vi "43 Config File Get Input Scales (x64-2018).vi"   [LabVIEW 2017]
uses:
  <vilib>/Utility/config.llb/Read Key (I32).vi
  24 Global Front Panel (x64-2018).vi
  <vilib>/Utility/config.llb/NI_LVConfig.lvlib
types:
  T1 = typedef "NI_LVConfig.lvlib/Config Data RefNum.ctl" = refnum<k1>
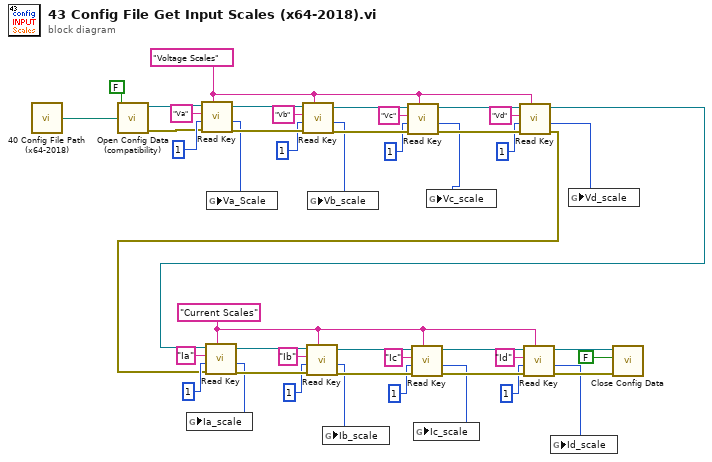
[diagram p0: block diagram]
diagram:
  w15 = "Current Scales" ("section")
  w16 = "Voltage Scales" ("section")
  n1 = call "40 Config File Path (x64-2018).vi"() -> ("Configuration File Path"=w9:path)
  n2 = call <vilib>:"Open Config Data (compatibility).vi"("create file if necessary (T)"=FALSE ("create file if necessary? (T)"), "configuration file path"=w9) -> ("error out"=w33:errorcluster, "refnum"=w32:T1)  [unwired: 7 in, 1 out]
  n3 = call-poly <vilib>:"Read Key.vi"("section"=w16, "error in (no error)"=w33, "default value"=1, "key"="Va", "refnum"=w32) -> ("error out"=w39:errorcluster, "value"=w8:i32, "refnum out"=w38:T1)  [unwired: 3 in, 1 out]
  n4 = global write "24 Global Front Panel (x64-2018).vi" "Va_Scale"(w8) -> ()
  n5 = call-poly <vilib>:"Read Key.vi"("section"=w16, "error in (no error)"=w39, "default value"=1, "key"="Vb", "refnum"=w38) -> ("error out"=w43:errorcluster, "value"=w7:i32, "refnum out"=w42:T1)  [unwired: 3 in, 1 out]
  n6 = global write "24 Global Front Panel (x64-2018).vi" "Vb_scale"(w7) -> ()
  n7 = call-poly <vilib>:"Read Key.vi"("section"=w16, "error in (no error)"=w43, "default value"=1, "key"="Vc", "refnum"=w42) -> ("error out"=w47:errorcluster, "value"=w6:i32, "refnum out"=w46:T1)  [unwired: 3 in, 1 out]
  n8 = global write "24 Global Front Panel (x64-2018).vi" "Vc_scale"(w6) -> ()
  n9 = call-poly <vilib>:"Read Key.vi"("section"=w16, "error in (no error)"=w47, "default value"=1, "key"="Vd", "refnum"=w46) -> ("error out"=w10:errorcluster, "value"=w5:i32, "refnum out"=w17:T1)  [unwired: 3 in, 1 out]
  n10 = call-poly <vilib>:"Read Key.vi"("section"=w15, "error in (no error)"=w10, "default value"=1, "key"="Ia", "refnum"=w17) -> ("error out"=w23:errorcluster, "value"=w4:i32, "refnum out"=w22:T1)  [unwired: 3 in, 1 out]
  n11 = global write "24 Global Front Panel (x64-2018).vi" "Ia_scale"(w4) -> ()
  n12 = call-poly <vilib>:"Read Key.vi"("section"=w15, "error in (no error)"=w23, "default value"=1, "key"="Ib", "refnum"=w22) -> ("error out"=w27:errorcluster, "value"=w3:i32, "refnum out"=w26:T1)  [unwired: 3 in, 1 out]
  n13 = global write "24 Global Front Panel (x64-2018).vi" "Ib_scale"(w3) -> ()
  n14 = call-poly <vilib>:"Read Key.vi"("section"=w15, "error in (no error)"=w27, "default value"=1, "key"="Ic", "refnum"=w26) -> ("error out"=w31:errorcluster, "value"=w2:i32, "refnum out"=w30:T1)  [unwired: 3 in, 1 out]
  n15 = global write "24 Global Front Panel (x64-2018).vi" "Ic_scale"(w2) -> ()
  n16 = call-poly <vilib>:"Read Key.vi"("section"=w15, "error in (no error)"=w31, "default value"=1, "key"="Id", "refnum"=w30) -> ("error out"=w13:errorcluster, "value"=w1:i32, "refnum out"=w14:T1)  [unwired: 3 in, 1 out]
  n17 = global write "24 Global Front Panel (x64-2018).vi" "Id_scale"(w1) -> ()
  n18 = global write "24 Global Front Panel (x64-2018).vi" "Vd_scale"(w5) -> ()
  n19 = call <vilib>:"Close Config Data.vi"("error in (no error)"=w13, "write file if changed (T)"=FALSE ("write configuration file? (T)"), "refnum"=w14) -> ()  [unwired: 7 in, 2 out]
